vi "Find_Beam_Max_Pos.vi"(3 "Mode":T7, 5 "Traverse line In":T4 {"Row Duration (mins)" format="%#.1f"; "Row No" min=0; "Trace Gas Concentration (%)" min=0.0 format="%#.2f"; "Emission Rate (l/min)" format="%#.2f"; "Tunnel Speed" format="%#.2f"; "Start X" format="%#.2f"; "Start Y" format="%#.2f"; "Start Z" format="%#.2f"; "End X" format="%#.2f"; "End Y" format="%#.2f"; "End Z" format="%#.2f"; "Averaging time (min)" min=0.0 format="%#.2f"}) -> (0 "Error Message":string, 1 "Status":T3, 2 "Traverse line Out":T4 {"Row Duration (mins)" format="%#.1f"; "Row No" min=0; "Trace Gas Concentration (%)" min=0.0 format="%#.2f"; "Emission Rate (l/min)" format="%#.2f"; "Tunnel Speed" format="%#.2f"; "Start X" format="%#.2f"; "Start Y" format="%#.2f"; "Start Z" format="%#.2f"; "End X" format="%#.2f"; "End Y" format="%#.2f"; "End Z" format="%#.2f"; "Averaging time (min)" min=0.0 format="%#.2f"})   [LabVIEW 2010]
uses:
  Gen Trav/Traverse_cluster.ctl
  Gen Trav/Spacing.ctl
  Controls/Multi_run_mode.ctl
  Controls/User_Specific_mode.ctl
  Gen Trav/Multi_Run_Status.ctl
  Controls/Beam_Type.ctl
  Gen Trav/Route mapping/Axis.ctl
  ADAM Client/Sub VIs/ADAM Controls/Remember_value_mode.ctl
  Globals/Meas_global.vi
  Utilities/Email_transfer_global.vi
panel:
  out "Picture Log":path
  out "First Call":bool
  out "Fixed Axis":T1
  out "Beams to find":T2[](array[typedef]) items=["Green Unshifted", "Green Shifted", "Blue Unshifted", "Blue Shifted"]
  out "Beam Data":dbl[][](array[numeric]) format="%.2f"
  out "Beam Type":T2 items=["Green Unshifted", "Green Shifted", "Blue Unshifted", "Blue Shifted"]
  # "X                Y                 Z        Datum Power"
  # "Green Unshifted\nGreen Shifted\nBlue Unshifted\nBlue Shifted"
  # "X           Y            Z"
  # "Start"
  # "End"
  # "X           Y            Z"
  # "Start"
  # "End"
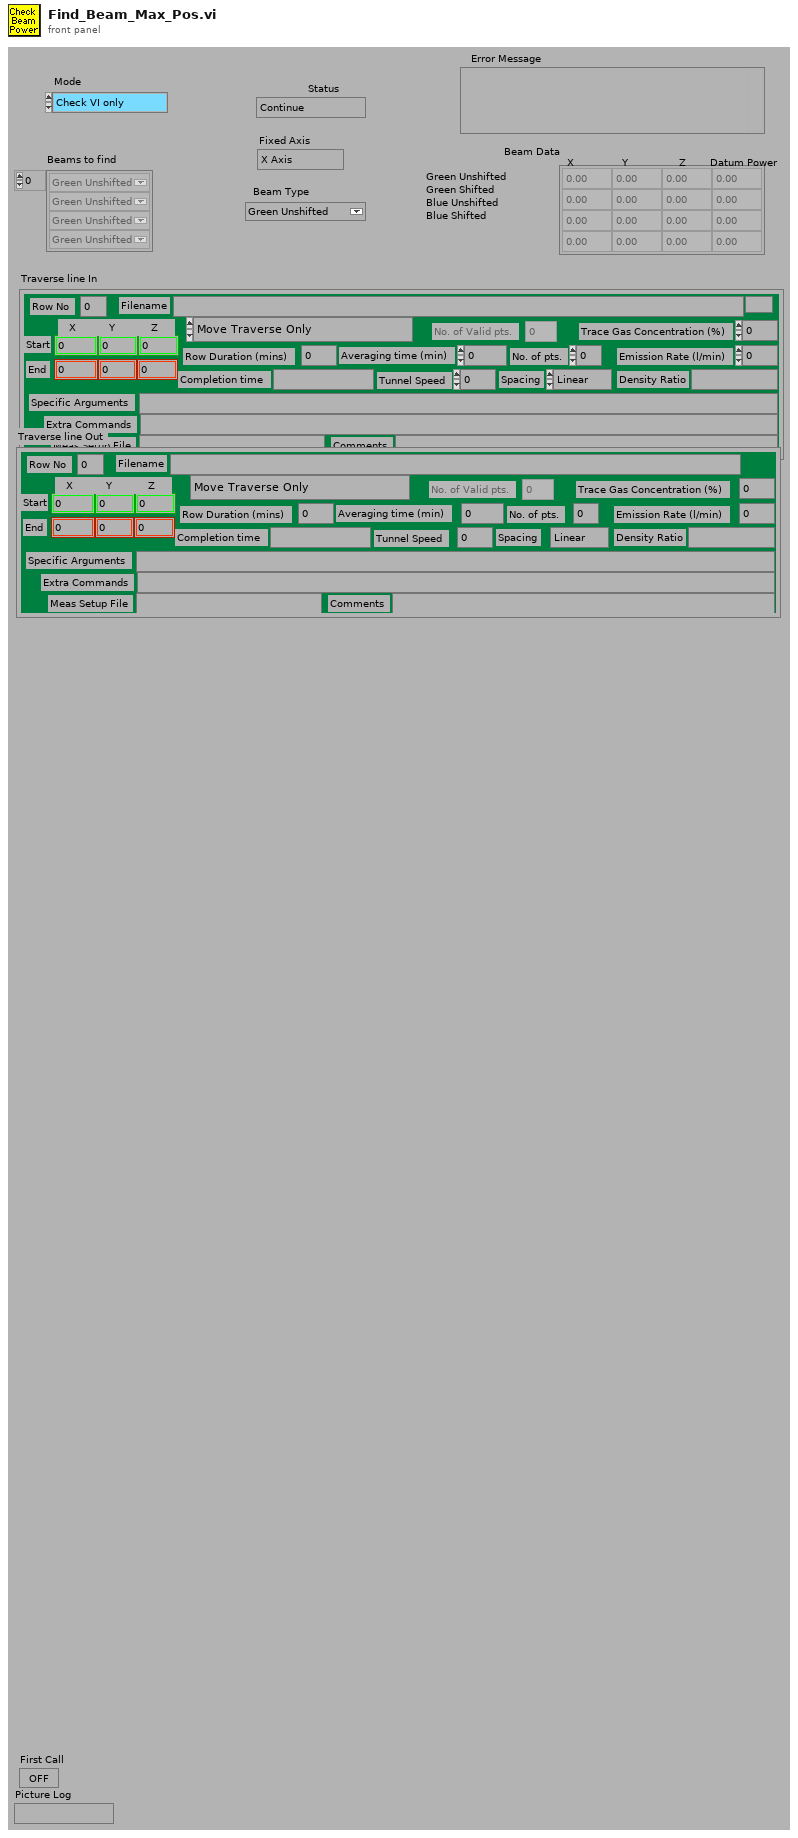
[diagram p1: front panel]
types:
  T1 = typedef "Axis.ctl" = enum16{"X Axis", "X Axis -ve", "Y Axis", "Y Axis -ve", "Z Axis", "Z Axis -ve"}
  T2 = typedef "Beam_Type.ctl" = u16
  T3 = typedef "Multi_Run_Status.ctl" = enum16{"Continue", "Jump to Next Point", "Jump to Next Row", "Jump To Fall Back", "Terminate Run"}
  T4 = typedef "Traverse_cluster.ctl" = cluster{"Start X":dbl, "Start Y":dbl, "Start Z":dbl, "End X":dbl, "End Y":dbl, "End Z":dbl, "No. of pts.":i32, "Spacing":T5, "Filename":path, "Tunnel Speed":dbl, "Averaging time (min)":dbl, "Extra Commands":string, "Specific Arguments":string, "Emission Rate (l/min)":dbl, "Trace Gas Concentration (%)":dbl, "Density Ratio":string, "Comments":string, "Row No":i32, "Row Type Selector":T6, "Completion time":string, "Row Duration (mins)":dbl, "No. of Valid pts.":i32, "Meas Setup File":string}
  T5 = typedef "Spacing.ctl" = enum16{"Linear", "Log", "Gauss", "Specified", "N/A"}
  T6 = typedef "Multi_run_mode.ctl" = enum16{"Move Traverse Only", "Set Tunnel Speed Only", "Set Source Only", "Set Measurement Conditions", "Single Measurement", "Vertical Profile", "Lateral Profile", "Longitudinal Profile", "Explore Volume", "Multi-Axis Profile", "Auto Calibrate", "Meas Fast FID Bkgnd", "Check Beam Power", "Scanning Valve Measurement", "Run VI Named:", "Set ADAM Ch", "Wait (minutes)", "Send Message", "Synchronize With:", "Fall Back to this Row", "Turn Off Row Repeating", "Blank Row"}
  T7 = typedef "User_Specific_mode.ctl" = enum16{"Check VI only", "Run VI"}
  T8 = typedef "Remember_value_mode.ctl" = enum16{"Read only", "Read and Write"}
  T9 = enum16{"Load From Excel File", "Save to Excel File"}
  T10 = cluster{"second":i32, "minute":i32, "hour":i32, "day of month":i32, "month":i32, "year":i32, "day of week":i32, "day of year":i32, "is DST":i32}
  T11 = cluster{"path":path, "data":string, "binary":bool, "MIME content-type \n(application/octet-stream)":string}[]
  T12 = cluster{"path":path, "data":string, "binary":bool, "MIME content-type \n(application/octet-stream)":string}
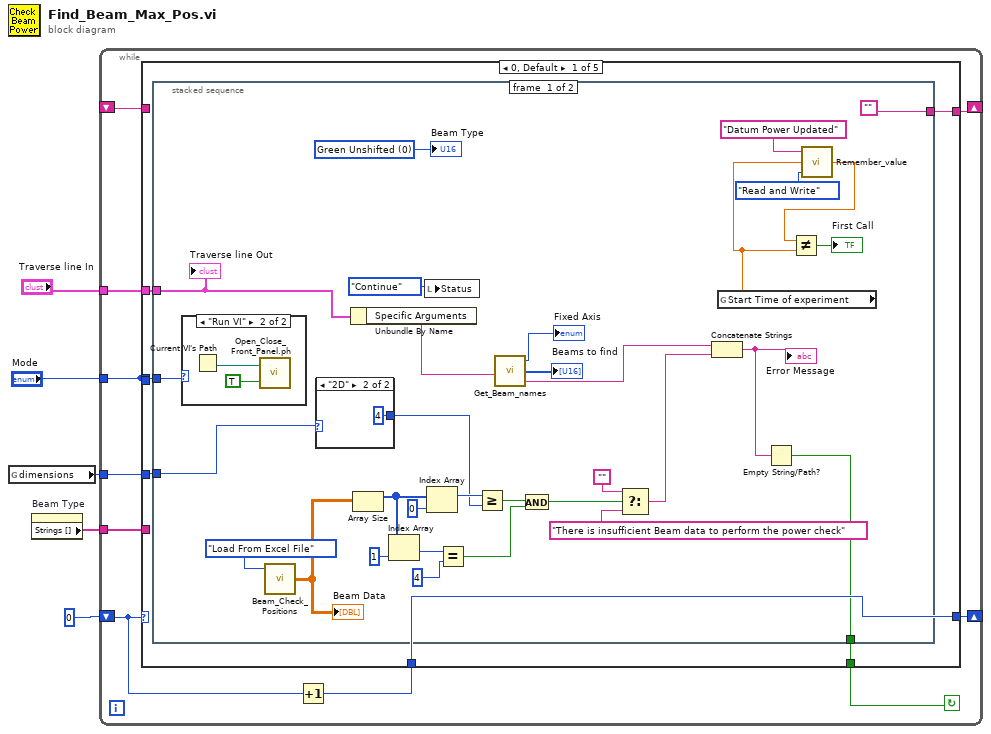
[diagram p0: block diagram]
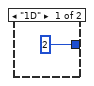
[diagram p2: hidden frame]
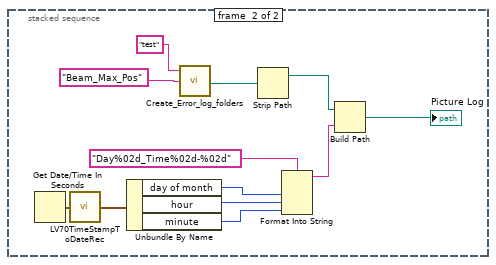
[diagram p4: hidden frame]
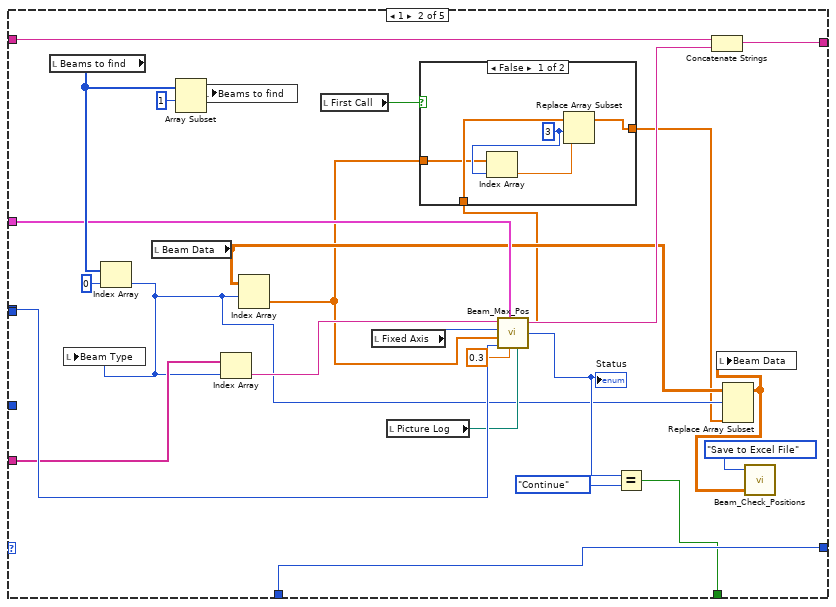
[diagram p5: hidden frame]
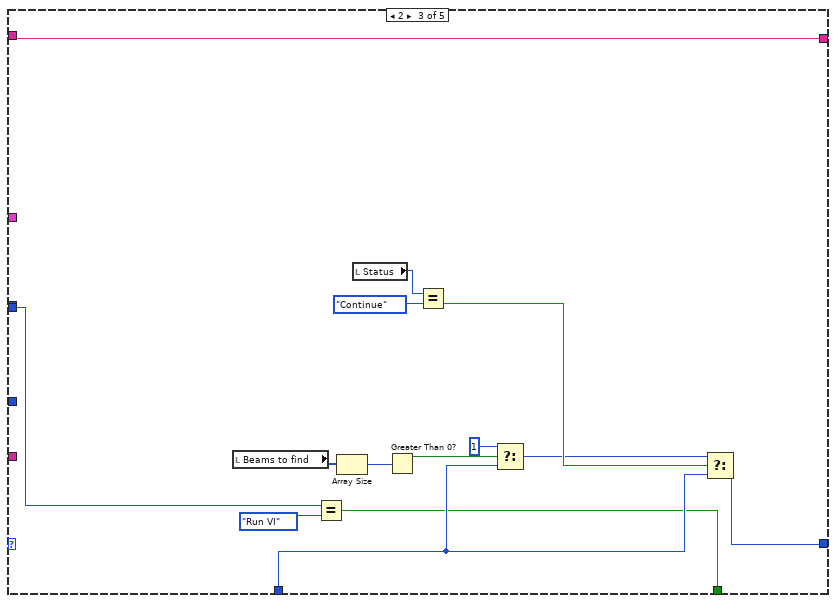
[diagram p7: hidden frame]
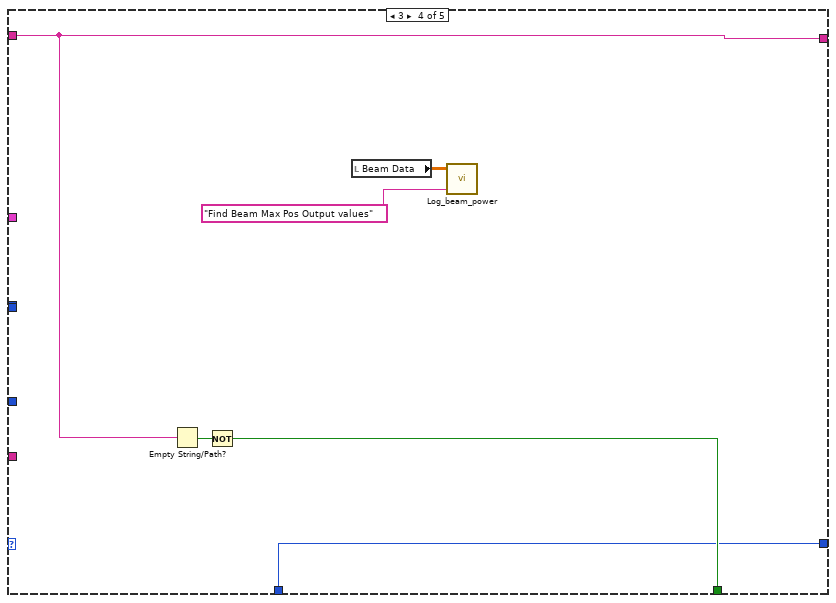
[diagram p8: hidden frame]
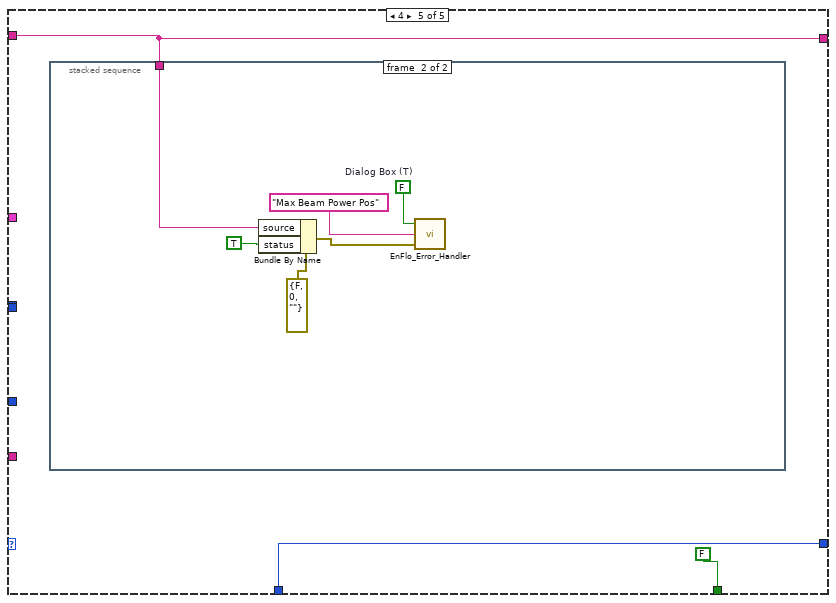
[diagram p9: hidden frame]
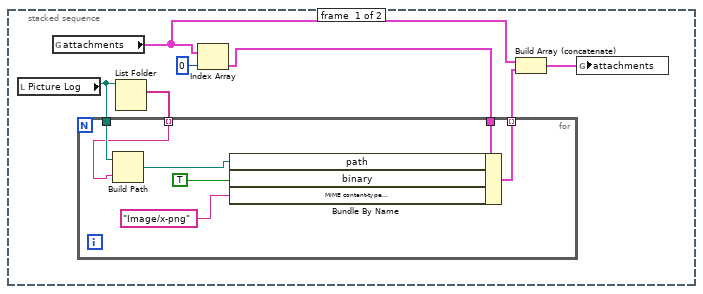
[diagram p10: hidden frame]
diagram:
  n1 = global read "Meas_global.vi" "dimensions"() -> (w1:enum16{"1D", "2D"})
  n2 = property on="Beam Type" class="Ring (strict)"() -> ("Strings []"=w2:string[])  [unwired: 2 in, 2 out]
  n3 = while {
    shift-left: _ -> [w6]
    shift-right: [w7] -> _
    tunnel: w1 -> [w9]
    tunnel: w2 -> [w13]
    tunnel: "Traverse line In" -> [w14]
    tunnel: "Mode" -> [w8]
    shift-left: 0 -> [w15]
    shift-right: [w10] -> _
    stop <- w12 continue-if-true
    n4 = Increment(x=w15) -> (x+1=w11:i32)
    n5 = case shown="0, Default" w15 {
      tunnel: w14 -> [w17 w88 _ _ _]
      tunnel: w8 -> [w20 w89 _ _ _]
      tunnel: w13 -> [_ w80 _ _ _]
      tunnel: [w18 w82 w107 w117 FALSE] -> w12
      tunnel: w11 -> [w21 w91 w111 w116 w124]
      tunnel: [w21 w91 w110 w116 w124] -> w10
      tunnel: w9 -> [w19 _ _ _ _]
      tunnel: w8 -> [_ _ w108 _ _]
      tunnel: [w16 w85 w102 w119 w122] -> w7
      tunnel: w6 -> [_ w87 w102 w119 w122]
      frame 0, Default {
        n6 = stacked-sequence {
          tunnel: w20 -> [w48 _]
          tunnel: w19 -> [w47 _]
          tunnel: [w40 _] -> w18
          tunnel: w17 -> [w32 _]
          tunnel: ["" _] -> w16
          frame #0 {
            w52 = T2 0 items=["Green Unshifted", "Green Shifted", "Blue Unshifted", "Blue Shifted"] ("Beam Type")
            n7 = case shown="\"Run VI\"" w48 {
              frame "Check VI only" {
              }
              frame "Run VI" {
                n8 = Current VI's Path() -> (path=w56:path)
                n9 = call "Open_Close_Front_Panel.ph.vi"("Front Panel Window:Open"=TRUE, "VI path"=w56) -> ()  [unwired: 2 out]
              }
            }
            n10 = call "Beam_Check_Positions.vi"("Mode"=T9."Load From Excel File") -> ("Values Out"=w50:dbl[][])  [unwired: 1 in, 1 out]
            "Beam Data" <- w50
            n11 = case shown="\"2D\"" w47 {
              tunnel: [2 4] -> w45
              frame "1D" {
              }
              frame "2D" {
              }
            }
            n12 = Unbundle By Name(w32) -> ("Specific Arguments"=w22:string)
            n13 = Array Size(array=w50) -> (size(s)=w38:i32[])
            n14 = Index Array(array=w38, index=1 ("Index")) -> (element=w37:i32)
            n15 = local write "Status"(Multi_Run_Status."Continue" ("Status")) -> ()
            n16 = Index Array(array=w38, index=0 ("Index")) -> (element=w46:i32)
            n17 = Equal?(x=w37, y=4) -> (x = y?=w34:bool)
            n18 = Greater Or Equal?(x=w46, y=w45) -> (x >= y?=w35:bool)
            n19 = call "Get_Beam_names.vi"("String Value"=w22) -> ("Fixed Axis"=→"Fixed Axis":T1, "Beam Array"=→"Beams to find":T2[], "Error Comments"=w31:string)
            n20 = And(x=w35, y=w34) -> (x .and. y?=w33:bool)
            n21 = Select(t="", s=w33, f="There is insufficient Beam data to perform the power check") -> (s? t:f=w42:string)
            n22 = Concatenate Strings(w31, w42) -> (w41:string)
            "Error Message" <- w41
            n23 = global read "Meas_global.vi" "Start Time of experiment"() -> (w25:dbl)
            n24 = Empty String/Path?(string/path=w41) -> (empty?=w40:bool)
            n25 = call "Remember_value.vi"("Mode"=Remember_value_mode."Read and Write", "Input Value"=w25, "Ch name"="Datum Power Updated") -> ("Output Value"=w26:dbl)
            n26 = Not Equal?(x=w26, y=w25) -> (x != y?=→"First Call":bool)
            "Beam Type" <- w52
            "Traverse line Out" <- w32
          }
          frame #1 {
            n27 = Get Date/Time In Seconds() -> (seconds since 1Jan1904=w58:timestamp)
            n28 = call <vilib>:"LV70TimeStampToDateRec.vi"("time stamp"=w58) -> ("date time rec"=w67:T10)
            n29 = Unbundle By Name(w67) -> ("day of month"=w64:i32, "hour"=w65:i32, "minute"=w66:i32)
            n30 = call "Create_Error_log_folders.vi"("Log Folder"="Beam_Max_Pos" ("name or relative path"), "Log Filename"="test") -> ("Server copy Location"=w60:path)  [unwired: 1 in, 2 out]
            n31 = Strip Path(path=w60) -> (stripped path=w68:path)  [unwired: 1 out]
            n32 = Format Into String(format string="Day%02d_Time%02d-%02d", w64, w65, w66) -> (resulting string=w69:string)  [unwired: 2 in, 1 out]
            n33 = Build Path(base path=w68, name or relative path=w69) -> (appended path=→"Picture Log":path)
          }
        }
      }
      frame 1 {
        n34 = local read "Beams to find"() -> (w94:T2[])
        n35 = Index Array(array=w94, index=0 ("Index")) -> (element=w77:T2)
        n36 = local write "Beam Type"(w77) -> ()
        n37 = local read "Beam Data"() -> (w78:dbl[][])
        n38 = Array Subset(array=w94, index=1 ("Array Index")) -> (w92:T2[])  [unwired: 1 in]
        n39 = local write "Beams to find"(w92) -> ()
        n40 = Index Array(array=w80, index=w77) -> (element=w79:string)
        n41 = Index Array(array=w78, index (row)=w77) -> (element=w71:dbl[])  [unwired: 1 in]
        n42 = local read "First Call"() -> (w76:bool)
        n43 = local read "Fixed Axis"() -> (w90:T1)
        n44 = local read "Picture Log"() -> (w81:path)
        n45 = call "Beam_Max_Pos.vi"("Picture Log"=w81, "Search Step (mm)"=0.3, "Mode"=w89, "Starting Position"=w71, "Traverse line In"=w88, "Fixed Axis"=w90, "Beam Name"=w79) -> ("Status"=w83:T3, "Beam maxima"=w74:dbl[], "Message"=w86:string)  [unwired: 1 out]
        "Status" <- w83
        n46 = case shown="False" w76 {
          tunnel: [w99 w101] -> w75
          tunnel: w74 -> [w100 w101]
          tunnel: w71 -> [w97 _]
          frame False {
            w98 = 3 ("index")
            n47 = Index Array(array=w97, index=w98) -> (element=w96:dbl)
            n48 = Replace Array Subset(array=w100, new element=w96, index=w98) -> (w99:dbl[])
          }
          frame True {
          }
        }
        n49 = Equal?(x=w83, y=Multi_Run_Status."Continue" ("Status")) -> (x = y?=w82:bool)
        n50 = Concatenate Strings(w87, w86) -> (w85:string)
        n51 = Replace Array Subset(array=w78, new element=w75, index (row)=w77) -> (w72:dbl[][])  [unwired: 1 in]
        n52 = local write "Beam Data"(w72) -> ()
        n53 = call "Beam_Check_Positions.vi"("Values"=w72, "Mode"=T9."Save to Excel File") -> ()  [unwired: 2 out]
      }
      frame 2 {
        n54 = local read "Beams to find"() -> (w106:T2[])
        n55 = Equal?(x=w108, y=User_Specific_mode."Run VI" ("Mode")) -> (x = y?=w107:bool)
        n56 = Array Size(array=w106) -> (size(s)=w105:i32)
        n57 = local read "Status"() -> (w115:T3)
        n58 = Greater Than 0?(x=w105) -> (x > 0?=w104:bool)
        n59 = Equal?(x=w115, y=Multi_Run_Status."Continue" ("Status")) -> (x = y?=w113:bool)
        n60 = Select(t=1, s=w104, f=w111) -> (s? t:f=w112:i32)
        n61 = Select(t=w112, s=w113, f=w111) -> (s? t:f=w110:i32)
      }
      frame 3 {
        n62 = Empty String/Path?(string/path=w119) -> (empty?=w118:bool)
        n63 = Not(x=w118) -> (.not. x?=w117:bool)
        n64 = local read "Beam Data"() -> (w121:dbl[][])
        n65 = call "Log_beam_power.vi"("Message"="Find Beam Max Pos Output values", "Beam Data"=w121) -> ()  [unwired: 4 out]
      }
      frame 4 {
        n66 = stacked-sequence {
          tunnel: w122 -> [_ w139]
          frame #0 {
            n67 = local read "Picture Log"() -> (w126:path)
            n68 = global read "Email_transfer_global.vi" "attachments"() -> (w129:T11)
            n69 = List Folder(path=w126) -> (filenames=w125:string[])  [unwired: 1 in, 5 out]
            n70 = Index Array(array=w129, index=0) -> (element=w128:T12)
            n71 = for {
              tunnel: [w136] -> w131 mode=indexing
              tunnel: w128 -> [w135]
              tunnel: w126 -> [w134]
              tunnel: w125 -> [w133] mode=indexing
              n72 = Build Path(base path=w134, name or relative path=w133) -> (appended path=w132:path)
              n73 = Bundle By Name(cluster=w135, "path"=w132, "binary"=TRUE, "MIME content-type \n(application/octet-stream)"="Image/x-png" ("MIME content-type \n(application/octet-stream)")) -> (w136:T12)
            }
            n74 = Build Array (concatenate)(w129, w131) -> (w130:T11)
            n75 = global write "Email_transfer_global.vi" "attachments"(w130) -> ()
          }
          frame #1 {
            w143 = FALSE  # Dialog Box (T)
            n76 = Bundle By Name(cluster=errorcluster {"status"=FALSE, "code"=0, "source"=""} ("error in (no error)"), "source"=w139, "status"=TRUE ("Bundle Element")) -> (w141:errorcluster)
            n77 = call "EnFlo_Error_Handler.vi"("error in (no error)"=w141, "Error Type"="Max Beam Power Pos", "Dialog Box (T)"=w143) -> ()  [unwired: 3 out]
          }
        }
      }
    }
  }
